vi "Read LVCAM.vi"(11 "Read LVCAM in":refnum<class "Read LVCAM.lvclass">) -> (2 "LVCAM":refnum<class "LVCAM.lvclass">)   [LabVIEW 2021, in "LVCAM.lvlib" / "Read LVCAM.lvclass"]
uses:
  Read LVCAM.lvclass
  LVCAM/LVCAM.lvclass
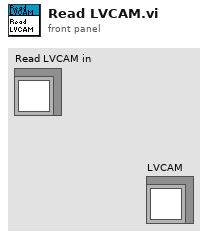
[diagram p1: front panel]
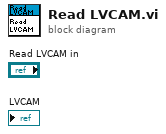
[diagram p0: block diagram]
diagram:
